vi "panel sizing.vi"(9 "Position In":T1, 11 "Size In":T2) -> (1 "Position Out":cluster{i32, i32}, 3 "Size Out":cluster{i32, i32})   [LabVIEW 2019]
uses:
  <vilib>/Utility/miscctls.llb/LVBoundsTypeDef.ctl
  <vilib>/Utility/miscctls.llb/LVPositionTypeDef.ctl
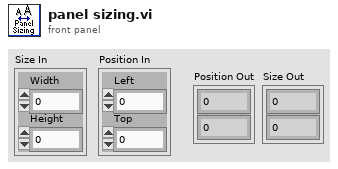
[diagram p1: front panel]
types:
  T1 = typedef "LVPositionTypeDef.ctl" = cluster{"Left":i32, "Top":i32}
  T2 = typedef "LVBoundsTypeDef.ctl" = cluster{"Width":u32, "Height":u32}
  T3 = typedef "LVRectTypeDef.ctl" = cluster{"Left":i16, "Top":i16, "Right":i16, "Bottom":i16}
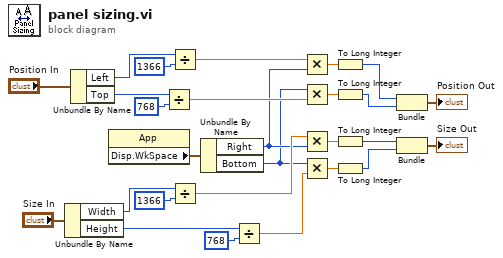
[diagram p0: block diagram]
diagram:
  n1 = Unbundle By Name("Size In") -> ("Width"=w17:u32, "Height"=w16:u32)
  n2 = Unbundle By Name("Position In") -> ("Left"=w13:i32, "Top"=w11:i32)
  n3 = property class="App"() -> ("Disp.WkSpace"=w27:T3)  [unwired: 2 in, 2 out]
  n4 = Divide(x=w11, y=768) -> (x/y=w9:dbl)
  n5 = Divide(x=w13, y=1366) -> (x/y=w10:dbl)
  n6 = Divide(x=w17, y=1366) -> (x/y=w22:dbl)
  n7 = Unbundle By Name(w27) -> ("Right"=w8:i16, "Bottom"=w7:i16)
  n8 = Divide(x=w16, y=768) -> (x/y=w24:dbl)
  n9 = Multiply(x=w10, y=w8) -> (x*y=w6:dbl)
  n10 = Multiply(x=w7, y=w9) -> (x*y=w5:dbl)
  n11 = Multiply(x=w22, y=w8) -> (x*y=w21:dbl)
  n12 = Multiply(x=w7, y=w24) -> (x*y=w23:dbl)
  n13 = To Long Integer(number=w6) -> (32bit integer=w4:i32)
  n14 = To Long Integer(number=w5) -> (32bit integer=w3:i32)
  n15 = To Long Integer(number=w21) -> (32bit integer=w20:i32)
  n16 = To Long Integer(number=w23) -> (32bit integer=w19:i32)
  n17 = Bundle(w4, w3) -> (→"Position Out":cluster{i32, i32})  [unwired: 1 in]
  n18 = Bundle(w20, w19) -> (→"Size Out":cluster{i32, i32})  [unwired: 1 in]
